vi "Remove SLSC Chassis.vi"(8 "error in (no error)":errorcluster, 9 "SLSC Chassis Name or IP":string, 10 "Target Name":string="Controller", 11 "SysDef in":refnum<k24>) -> (0 "error out":errorcluster, 1 "Removed":bool, 3 "SysDef out":refnum<k24>)   [LabVIEW 2020, in "VeriStand SLSC Scripting.lvlib"]
uses:
  VeriStand SLSC Scripting.lvlib
  NationalInstruments.VeriStand.SystemDefinitionAPI
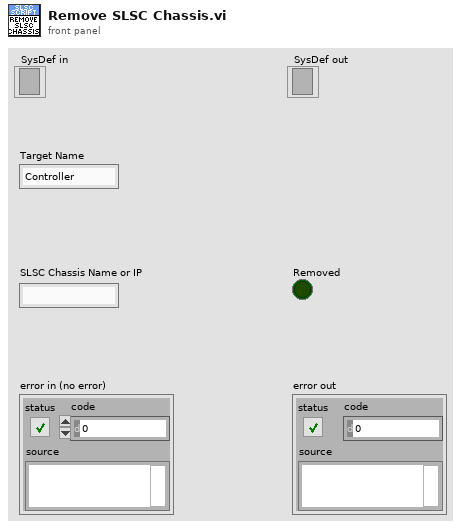
[diagram p1: front panel]
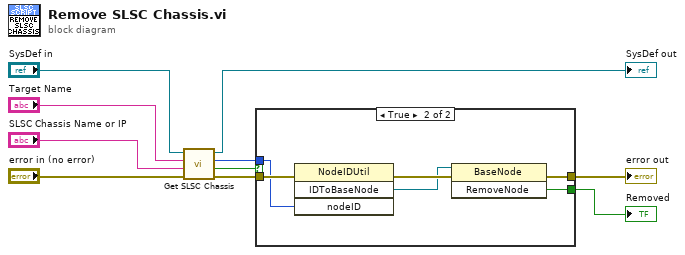
[diagram p0: block diagram]
diagram:
  n1 = call "Get SLSC Chassis.vi"("error in (no error)"="error in (no error)", "SLSC Chassis Name or IP"="SLSC Chassis Name or IP", "Target Name"="Target Name", "SysDef in"="SysDef in") -> ("error out"=w6:errorcluster, "Found"=w5:bool, "SLSC Chassis"=w4:u64, "SysDef out"=→"SysDef out":refnum<k24>)  [unwired: 4 in]
  n2 = case shown="True" w5 {
    tunnel: w6 -> [w11 w17]
    tunnel: w4 -> [_ w16]
    tunnel: [_ w13] -> w2
    tunnel: [w11 w12] -> w3
    frame False {
    }
    frame True {
      n3 = invoke class="NodeIDUtil" method="IDToBaseNode"(error in=w17, "nodeID"=w16) -> (error out=w15:errorcluster, "IDToBaseNode"=w14:refnum<k24>)  [unwired: 2 in, 2 out]
      n4 = invoke class="BaseNode" method="RemoveNode"(reference=w14, error in=w15) -> (error out=w12:errorcluster, "RemoveNode"=w13:bool)  [unwired: 1 in, 1 out]
    }
  }
  "error out" <- w3
  "Removed" <- w2
